vi "RPC Method GreeterService GetFeature.vi"(3 "error in (no error)":errorcluster, 4 "gRPCid in":T1, 5 "ServiceClass in":refnum<class "GreeterServiceImpl.lvclass">) -> (0 "error out":errorcluster, 1 "gRPCid out":T1, 2 "ServiceClass out":refnum<class "GreeterServiceImpl.lvclass">)   [LabVIEW 2019, in "UserCode_impl_server.lvlib" / "GreeterServiceImpl.lvclass"]
uses:
  GreeterServiceImpl.lvclass
  <vilib>/gRPC/LabVIEW gRPC Library/Shared/grpcId.ctl
  Generated_stub_server/RPC Messages/Greeter_res.ctl
  Generated_stub_server/RPC Messages/Greeter_res_res_oneof/Greeter_res_res_oneof.lvclass
  Generated_stub_server/RPC Messages/Greeter_req_req_oneof/Greeter_req_req_oneof.lvclass/Greeter_req_req_oneof.ctl
  Generated_stub_server/RPC Messages/Greeter_res_res_oneof/Greeter_res_res_oneof.lvclass/Greeter_res_res_oneof.ctl
  Generated_stub_server/Generated_stub_server.lvlib
  Generated_stub_server/RPC Messages/Greeter_req_req_oneof/Greeter_req_req_oneof.lvclass
  Generated_stub_server/RPC Service/GreeterServiceStub/GreeterServiceStub.lvclass
  <vilib>/gRPC/LabVIEW gRPC Library/grpc-lvsupport-release.lvlib
panel:
  out "gRPCid out 2":T1
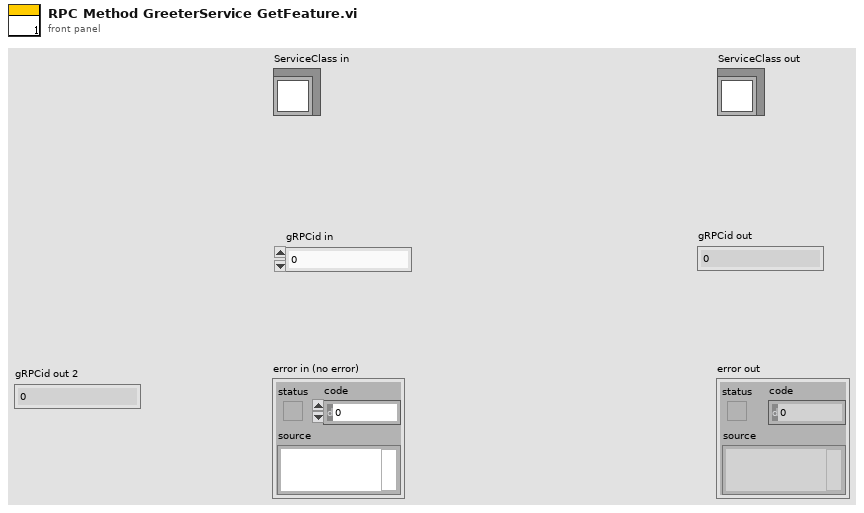
[diagram p1: front panel]
types:
  T1 = typedef "grpc-lvsupport-release.lvlib/grpcId.ctl" = u64
  T2 = typedef "Generated_stub_server.lvlib/Greeter_res.ctl" = cluster{"res_latitude":i32, "Greeter_res_res_oneof":refnum<class "Greeter_res_res_oneof.lvclass">}
  T3 = typedef "Generated_stub_server.lvlib/Greeter_req.ctl" = cluster{"req_latitude":i32, "Greeter_req_req_oneof":refnum<class "Greeter_req_req_oneof.lvclass">}
  T4 = typedef "Generated_stub_server.lvlib/Greeter_Color.ctl" = enum32{"RED", "GREEN", "BLUE"}
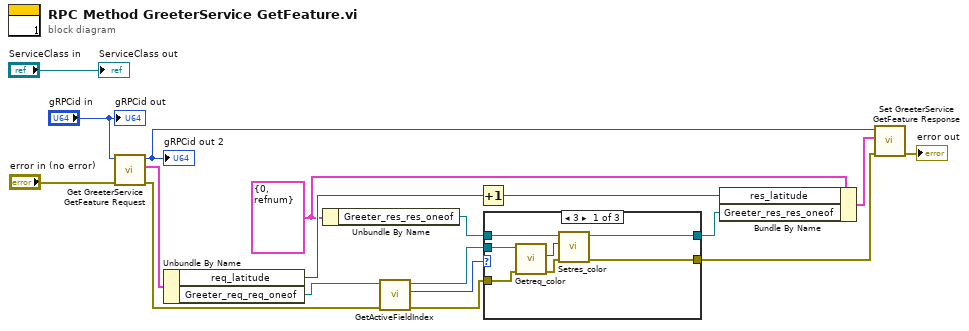
[diagram p0: block diagram]
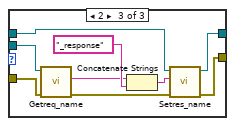
[diagram p3: hidden frame]
diagram:
  w8 = T2 {"res_latitude"=0, "Greeter_res_res_oneof"=refnum} ("Message Data")
  n1 = call "Get GreeterService GetFeature Request.vi"("error in (no error)"="error in (no error)", "gRPCid"="gRPCid in") -> ("error out"=w10:errorcluster, "Message Data"=w18:T3, "gRPCid out"=w5:T1)  [unwired: 7 in]
  "gRPCid out 2" <- w5
  n2 = Unbundle By Name(w18) -> ("req_latitude"=w17:i32, "Greeter_req_req_oneof"=w15:refnum<class "Greeter_req_req_oneof.lvclass">)
  n3 = Unbundle By Name(w8) -> ("Greeter_res_res_oneof"=w13:refnum<class "Greeter_res_res_oneof.lvclass">)
  n4 = call "GetActiveFieldIndex.vi"("error in (no error)"=w10, "OneOfTemplate in"=w15) -> ("error out"=w11:errorcluster, "Active Field Index"=w14:i32, "OneOfTemplate out"=w12:refnum<class "Greeter_req_req_oneof.lvclass">)  [unwired: 7 in]
  n5 = Increment(x=w17) -> (x+1=w16:i32)
  n6 = case shown="3" w14 {
    tunnel: w13 -> [w22 w27 w30]
    tunnel: w12 -> [w24 _ w36]
    tunnel: w11 -> [w25 w26 w35]
    tunnel: [w21 w27 w29] -> w9
    tunnel: [w20 w26 w28] -> w6
    frame 3 {
      n7 = call "Getreq_color.vi"("error in (no error)"=w25, "OneOfTemplate in"=w24) -> ("error out"=w23:errorcluster, "Get_Val"=w19:T4)  [unwired: 7 in, 1 out]
      n8 = call "Setres_color.vi"("error in (no error)"=w23, "Set_Val"=w19, "OneOfTemplate in"=w22) -> ("error out"=w20:errorcluster, "OneOfTemplate out"=w21:refnum<class "Greeter_res_res_oneof.lvclass">)  [unwired: 7 in]
    }
    frame Default {
    }
    frame 2 {
      n9 = call "Getreq_name.vi"("error in (no error)"=w35, "OneOfTemplate in"=w36) -> ("error out"=w34:errorcluster, "Get_Val"=w32:string)  [unwired: 7 in, 1 out]
      n10 = Concatenate Strings(w32, "_response" ("string")) -> (w31:string)
      n11 = call "Setres_name.vi"("error in (no error)"=w34, "Set_Val"=w31, "OneOfTemplate in"=w30) -> ("error out"=w28:errorcluster, "OneOfTemplate out"=w29:refnum<class "Greeter_res_res_oneof.lvclass">)  [unwired: 7 in]
    }
  }
  n12 = Bundle By Name(cluster=w8, "res_latitude"=w16, "Greeter_res_res_oneof"=w9) -> (w7:T2)
  n13 = call "Set GreeterService GetFeature Response.vi"("error in (no error)"=w6, "Message Data"=w7, "gRPCid in"=w5) -> ("error out"=→"error out":errorcluster)  [unwired: 8 in]
  "ServiceClass out" <- "ServiceClass in"
  "gRPCid out" <- "gRPCid in"
